vi "Unbundle.vi"(0 "index":i32, 5 "Commands Out Array":T1[](array[typedef])) -> (4 "Command":string, 6 "Time":string, 8 "Indicator1":bool, 10 "Indicator2":bool, 15 "Indicator3":bool)   [LabVIEW 2020]
uses:
  Controls/CLD 8 Data Cluster.ctl
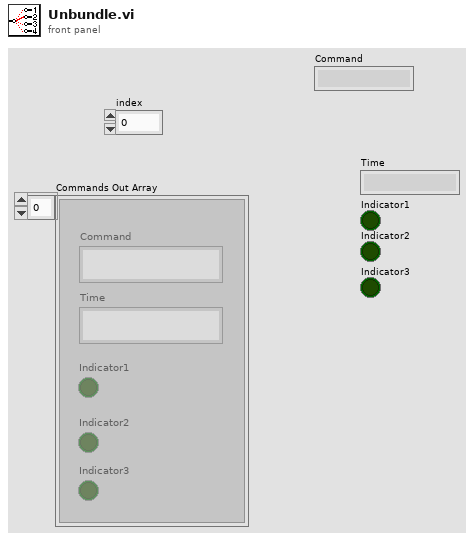
[diagram p1: front panel]
types:
  T1 = typedef "CLD 8 Data Cluster.ctl" = cluster{"Command":string, "Time":string, "Indicator1":bool, "Indicator2":bool, "Indicator3":bool}
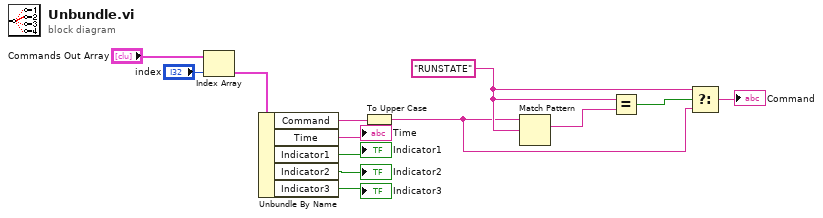
[diagram p0: block diagram]
diagram:
  w3 = "RUNSTATE" ("format string")
  n1 = Index Array(array="Commands Out Array", index="index") -> (element=w9:T1)
  n2 = Unbundle By Name(w9) -> ("Command"=w6:string, "Time"=→"Time":string, "Indicator1"=→"Indicator1":bool, "Indicator2"=→"Indicator2":bool, "Indicator3"=→"Indicator3":bool)
  n3 = To Upper Case(1:w6) -> (0:w2:string)
  n4 = Match Pattern(string=w2, regular expression=w3) -> (match substring=w5:string)  [unwired: 1 in, 3 out]
  n5 = Equal?(x=w3, y=w5) -> (x = y?=w4:bool)
  n6 = Select(t=w3, s=w4, f=w2) -> (s? t:f=→"Command":string)
